vi "update_status_line.vi"(7 "user event":refnum<user-event>, 10 "error in (no error)":errorcluster, 11 "message":string) -> (2 "error out":errorcluster, 3 "user event out":refnum<user-event>)   [LabVIEW 2016]
uses:
  Typedef/event var.ctl
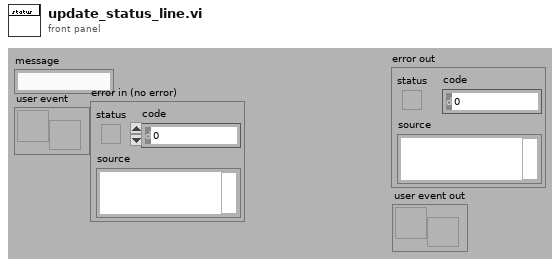
[diagram p1: front panel]
types:
  T1 = typedef "event var.ctl" = cluster{"Action":enum16{"Idle", "Update_comm_vars", "DMM_add_data", "Comm_add_data", "Therm_add_data", "Power_add_data", "Update graph", "Write log", "Setup and initialize", "Update Timing vars", "Update status line", "Update config refs"}, "Variant":variant}
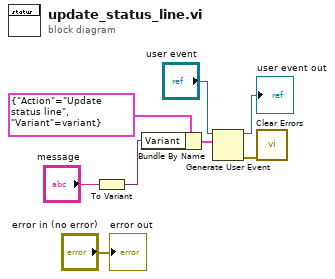
[diagram p0: block diagram]
diagram:
  n1 = To Variant(anything="message") -> (Variant=w8:variant)
  n2 = Bundle By Name(cluster=T1 {"Action"=enum."Update status line", "Variant"=variant} ("event data"), "Variant"=w8) -> (w7:T1)
  n3 = Generate User Event(user event="user event", event data cluster=w7) -> (user event out=→"user event out":refnum<user-event>, error out=w1:errorcluster)  [unwired: 2 in]
  n4 = call <vilib>:"Clear Errors.vi"("error in (no error)"=w1) -> ()  [unwired: 5 in, 2 out]
  "error out" <- "error in (no error)"
